vi "SM Update UI State.vi"(8 "error in (no error)":errorcluster, 10 "State":T1=enum."Initialising", 11 "Message Queue In":refnum<class "Delacor_lib_QMH_Message Queue.lvclass">) -> (0 "error out":errorcluster, 3 "Message Queue Out":refnum<class "Delacor_lib_QMH_Message Queue.lvclass">)   [LabVIEW 2020, in "StateMachine.lvlib" / "HSE-State-Machine.lvlib"]
doc: "Propagate state change to UI.\n\nHSE: This is only a place holder, in DQMH modules this would use the Message Queue. Implement your own communication mechanism here.\n____\nHAMPEL SOFTWARE ENGINEERING v2.6.0 (2023-12-19 10:54)"
uses:
  HSE-State-Machine.lvlib
  SM_States.ctl
  <vilib>/Delacor/Delacor QMH/Libraries/Message Queue_class/Delacor_lib_QMH_Message Queue.lvclass
  <vilib>/Delacor/Delacor QMH/Libraries/Message Queue_class/Delacor_lib_QMH_Message Queue.lvclass/Delacor_lib_QMH_Message Queue.ctl
  <vilib>/Delacor/Delacor QMH/Libraries/Message Queue_class/Delacor_lib_QMH_Enqueue Message (Single).vi
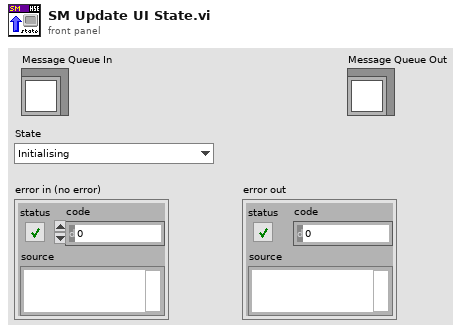
[diagram p1: front panel]
types:
  T1 = typedef "StateMachine.lvlib/HSE-State-Machine.lvlib/SM_States.ctl" = enum16{"No State - Error", "Error - Waiting For Action", "Initialising", "Standing by (idle)", "Waiting for External Trigger", "Polling for Signal Change", "Exiting"}
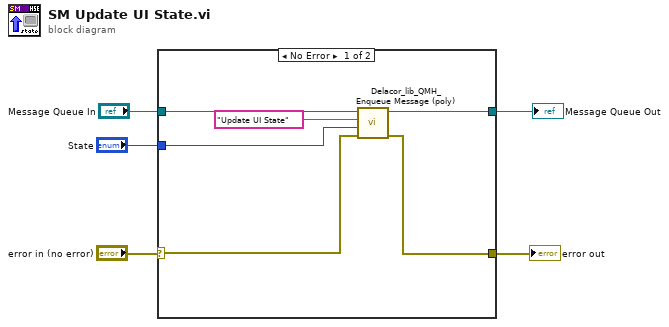
[diagram p0: block diagram]
diagram:
  n1 = case shown="No Error" "error in (no error)" {
    selector: "error in (no error)" -> [w9 w13]
    tunnel: [w8 w13] -> w4
    tunnel: "State" -> [w6 _]
    tunnel: [w10 w12] -> w2
    tunnel: "Message Queue In" -> [w11 w12]
    frame No Error {
      n2 = call-poly <vilib>:"Delacor_lib_QMH_Enqueue Message (poly).vi"("error in"=w9, "Message Data"=w6, "Message"="Update UI State", "Message Queue in"=w11) -> ("error out"=w8:errorcluster, "Message Queue out"=w10:refnum<class "Delacor_lib_QMH_Message Queue.lvclass">)  [unwired: 6 in]
    }
    frame Error {
    }
  }
  "error out" <- w4
  "Message Queue Out" <- w2
